vi "Pre-Build Custom Action.vi"(10 "Variant":variant) -> (0 "error out":errorcluster)   [LabVIEW 2017]
uses:
  <vilib>/Utility/traverseref.llb/TRef TravTarget.ctl
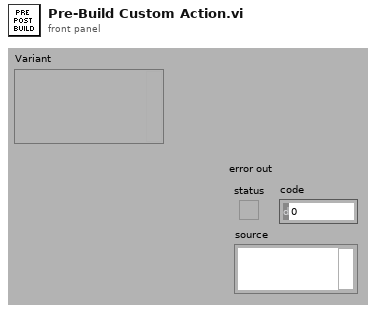
[diagram p1: front panel]
types:
  T1 = typedef "TRef TravTarget.ctl" = enum16{"FP", "BD", "Other"}
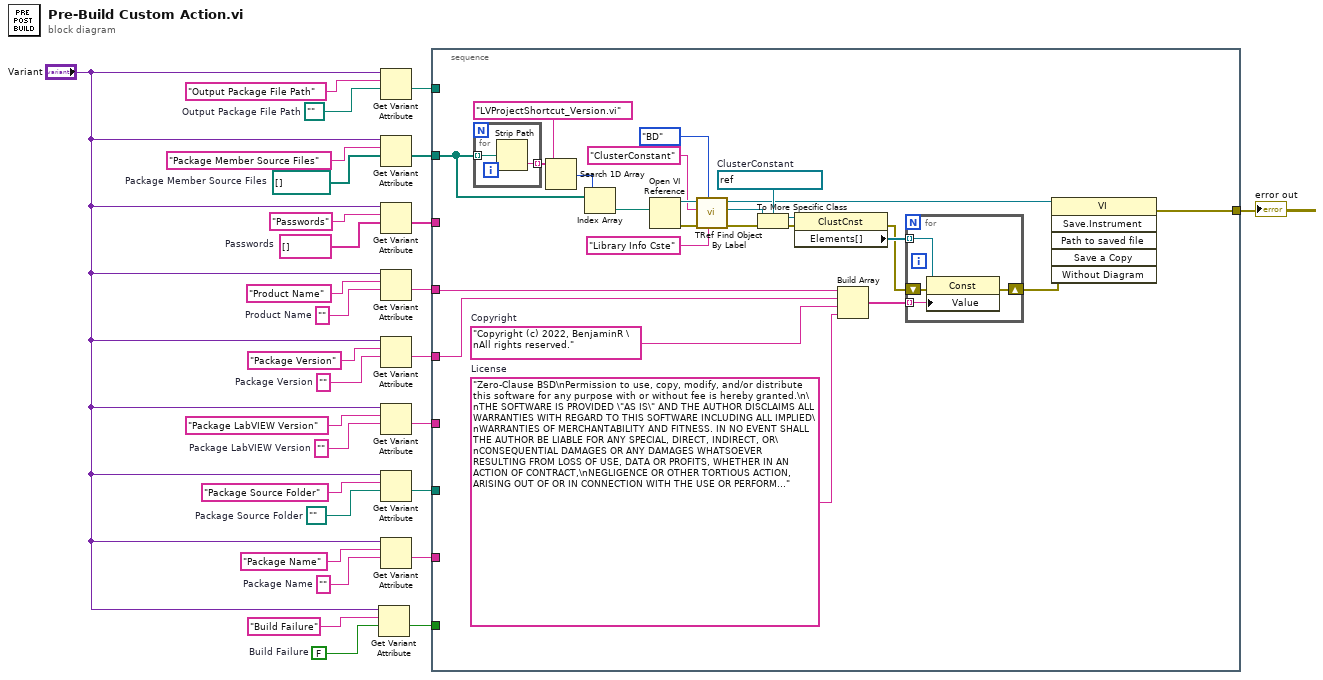
[diagram p0: block diagram]
diagram:
  w4 = FALSE  # Build Failure
  w14 = path ""  # Package Source Folder
  w15 = ""  # Package Name
  w18 = ""  # Package LabVIEW Version
  w20 = ""  # Package Version
  w22 = ""  # Product Name
  w24 = string[] []  # Passwords
  w26 = path[] []  # Package Member Source Files
  w28 = path ""  # Output Package File Path
  n1 = Get Variant Attribute(Variant="Variant", name="Build Failure", default value (empty Variant)=w4) -> (value=w2:bool)  [unwired: 1 in, 3 out]
  n2 = Get Variant Attribute(Variant="Variant", name="Output Package File Path", default value (empty Variant)=w28) -> (value=w13:path)  [unwired: 1 in, 3 out]
  n3 = Get Variant Attribute(Variant="Variant", name="Package Member Source Files", default value (empty Variant)=w26) -> (value=w12:path[])  [unwired: 1 in, 3 out]
  n4 = Get Variant Attribute(Variant="Variant", name="Passwords", default value (empty Variant)=w24) -> (value=w11:string[])  [unwired: 1 in, 3 out]
  n5 = Get Variant Attribute(Variant="Variant", name="Product Name", default value (empty Variant)=w22) -> (value=w10:string)  [unwired: 1 in, 3 out]
  n6 = Get Variant Attribute(Variant="Variant", name="Package Version", default value (empty Variant)=w20) -> (value=w9:string)  [unwired: 1 in, 3 out]
  n7 = Get Variant Attribute(Variant="Variant", name="Package LabVIEW Version", default value (empty Variant)=w18) -> (value=w8:string)  [unwired: 1 in, 3 out]
  n8 = Get Variant Attribute(Variant="Variant", name="Package Source Folder", default value (empty Variant)=w14) -> (value=w7:path)  [unwired: 1 in, 3 out]
  n9 = Get Variant Attribute(Variant="Variant", name="Package Name", default value (empty Variant)=w15) -> (value=w6:string)  [unwired: 1 in, 3 out]
  n10 = stacked-sequence {
    tunnel: w13 -> [_]
    tunnel: w12 -> [w52]
    tunnel: w11 -> [_]
    tunnel: w10 -> [w38]
    tunnel: w9 -> [w37]
    tunnel: w8 -> [_]
    tunnel: w7 -> [_]
    tunnel: w6 -> [_]
    tunnel: w2 -> [_]
    tunnel: [w30] -> w1
    frame #0 {
      w34 = "Copyright (c) 2022, BenjaminR \nAll rights reserved."  # Copyright
      w35 = "Zero-Clause BSD\nPermission to use, copy, modify, and/or distribute this software for any purpose with or without fee is hereby granted.\n\nTHE SOFTWARE IS PROVIDED \"AS IS\" AND THE AUTHOR DISCLAIMS ALL WARRANTIES WITH REGARD TO THIS SOFTWARE INCLUDING ALL IMPLIED\nWARRANTIES OF MERCHANTABILITY AND FITNESS. IN NO EVENT SHALL THE AUTHOR BE LIABLE FOR ANY SPECIAL, DIRECT, INDIRECT, OR\nCONSEQUENTIAL DAMAGES OR ANY DAMAGES WHATSOEVER RESULTING FROM LOSS OF USE, DATA OR PROFITS, WHETHER IN AN ACTION OF CONTRACT,\nNEGLIGENCE OR OTHER TORTIOUS ACTION, ARISING OUT OF OR IN CONNECTION WITH THE USE OR PERFORMANCE OF THIS SOFTWARE."  # License
      w42 = refnum<vi> refnum  # ClusterConstant
      n11 = for {
        tunnel: w52 -> [w60] mode=indexing
        tunnel: [w59] -> w54 mode=indexing
        n12 = Strip Path(path=w60) -> (name=w59:string)  [unwired: 1 out]
      }
      n13 = Search 1D Array(1D array=w54, element="LVProjectShortcut_Version.vi") -> (index of element=w51:i32)  [unwired: 1 in]
      n14 = Index Array(array=w52, index=w51) -> (element=w50:path)
      n15 = Open VI Reference(vi path=w50) -> (vi reference=w49:refnum<vi>, error out=w45:errorcluster)  [unwired: 5 in]
      n16 = call <vilib>:"TRef Find Object By Label.vi"("Label"="Library Info Cste", "Traverse Target"=TRef_TravTarget."BD", "error in (no error)"=w45, "Class Name"="ClusterConstant", "VI Ref"=w49) -> ("error out"=w43:errorcluster, "Found Obj Ref"=w44:refnum<vi>, "dup VI Ref"=w32:refnum<vi>)  [unwired: 3 in, 1 out]
      n17 = To More Specific Class(target class=w42, reference=w44, error in=w43) -> (specific class reference=w41:refnum<vi>, error out=w40:errorcluster)
      n18 = property class="ClustCnst"(reference=w41, error in=w40) -> (error out=w33:errorcluster, "Elements[]"=w39:refnum<vi>[])  [unwired: 1 out]
      n19 = Build Array(w38, w37, w34, w35) -> (w36:string[])
      n20 = for {
        tunnel: w39 -> [w58] mode=indexing
        tunnel: w36 -> [w57] mode=indexing
        shift-right: [w55] -> w31
        shift-left: w33 -> [w56]
        n21 = property class="Const"(reference=w58, error in=w56, "Value"=w57) -> (error out=w55:errorcluster)  [unwired: 1 out]
      }
      n22 = invoke class="VI" method="Save.Instrument"(reference=w32, error in=w31) -> (error out=w30:errorcluster)  [unwired: 4 in, 5 out]
    }
  }
  "error out" <- w1
